vi "write delete child queue message.vi"(11 "child":refnum<class "identifying queue.lvclass">) -> (3 "message":refnum<class "communicator message.lvclass">)   [LabVIEW 2015, in "communicator.lvclass"]
uses:
  communicator.lvclass
  message/communicator message.lvclass
  communicator queue/identifying queue.lvclass
  message/communicator message.lvclass/communicator message.ctl
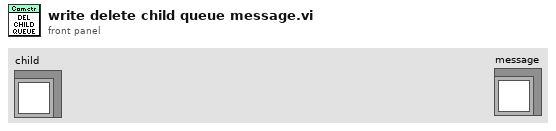
[diagram p1: front panel]
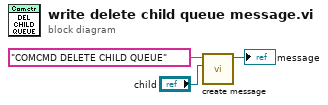
[diagram p0: block diagram]
diagram:
  n1 = call "create message.vi"("data"="child", "ID"="COMCMD DELETE CHILD QUEUE") -> ("message"=→"message":refnum<class "communicator message.lvclass">)  [unwired: 9 in]
